vi "Login.vi"() -> ()   [LabVIEW 2020, in "User Lib.lvlib"]
uses:
  User Lib.lvlib
  Database Lib.lvlib
panel:
  out "Error out 2":errorcluster
  out "Error out":errorcluster
  in  "Remember Me":bool
  in  "Cancel":bool
  in  "OK":bool
  in  "Password":string
  in  "Username":string
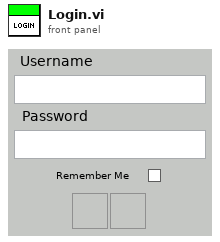
[diagram p1: front panel]
types:
  T1 = cluster{"date/time string":string, "date/time string":string, "code":i32, "date/time string":string, "source":string}
  T2 = cluster{i16, "date/time string":string, "date/time string":string, "Value":string, "Value":string}
  T3 = cluster{i32, "date/time string":string, "date/time string":string, string}
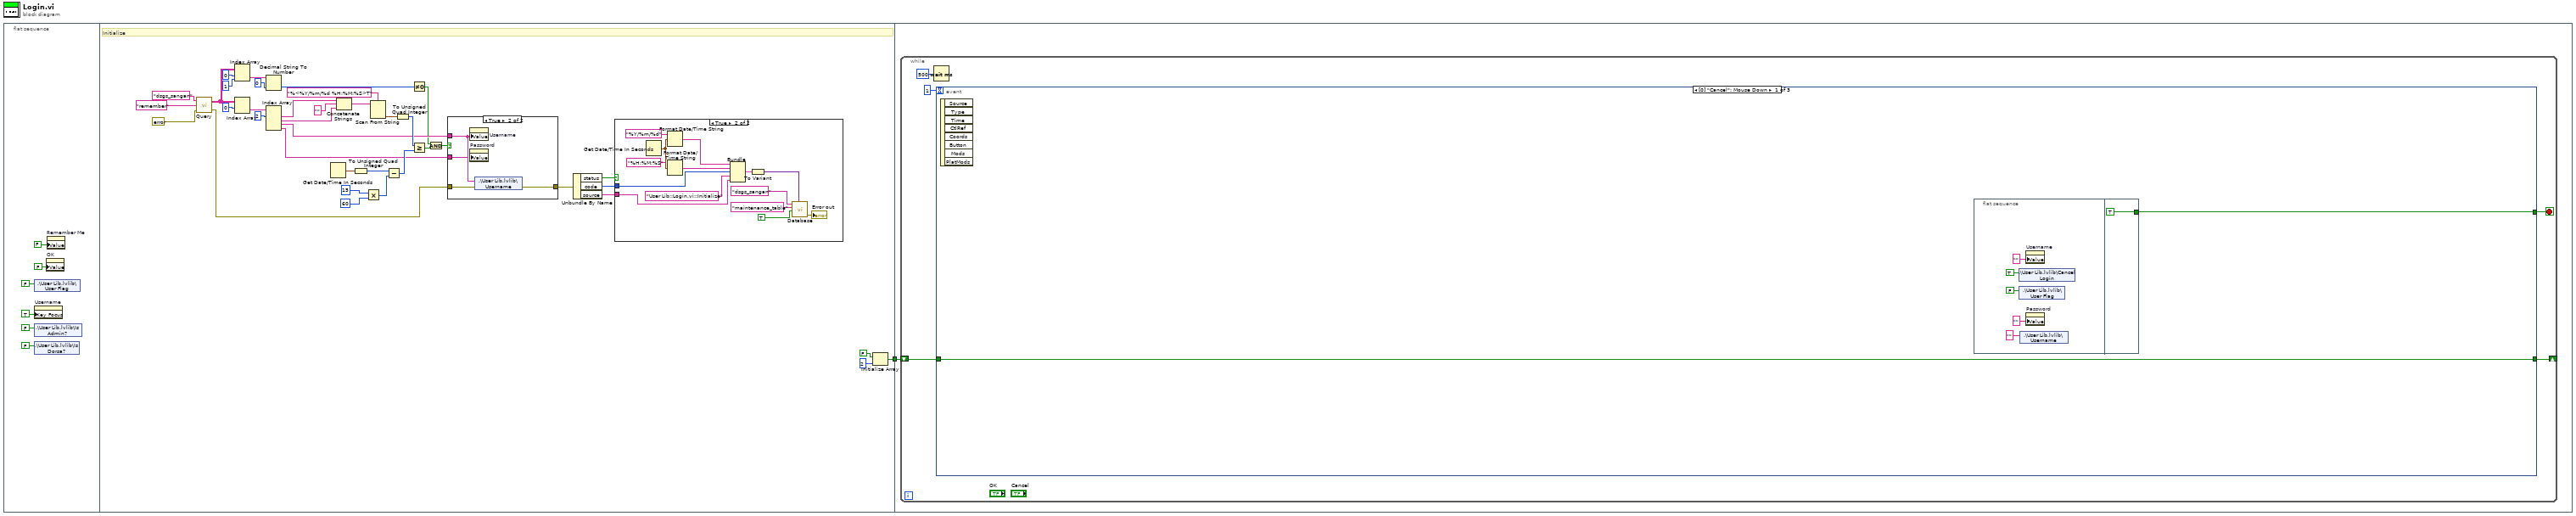
[diagram p0: block diagram]
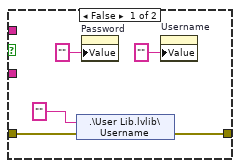
[diagram p3: hidden frame]
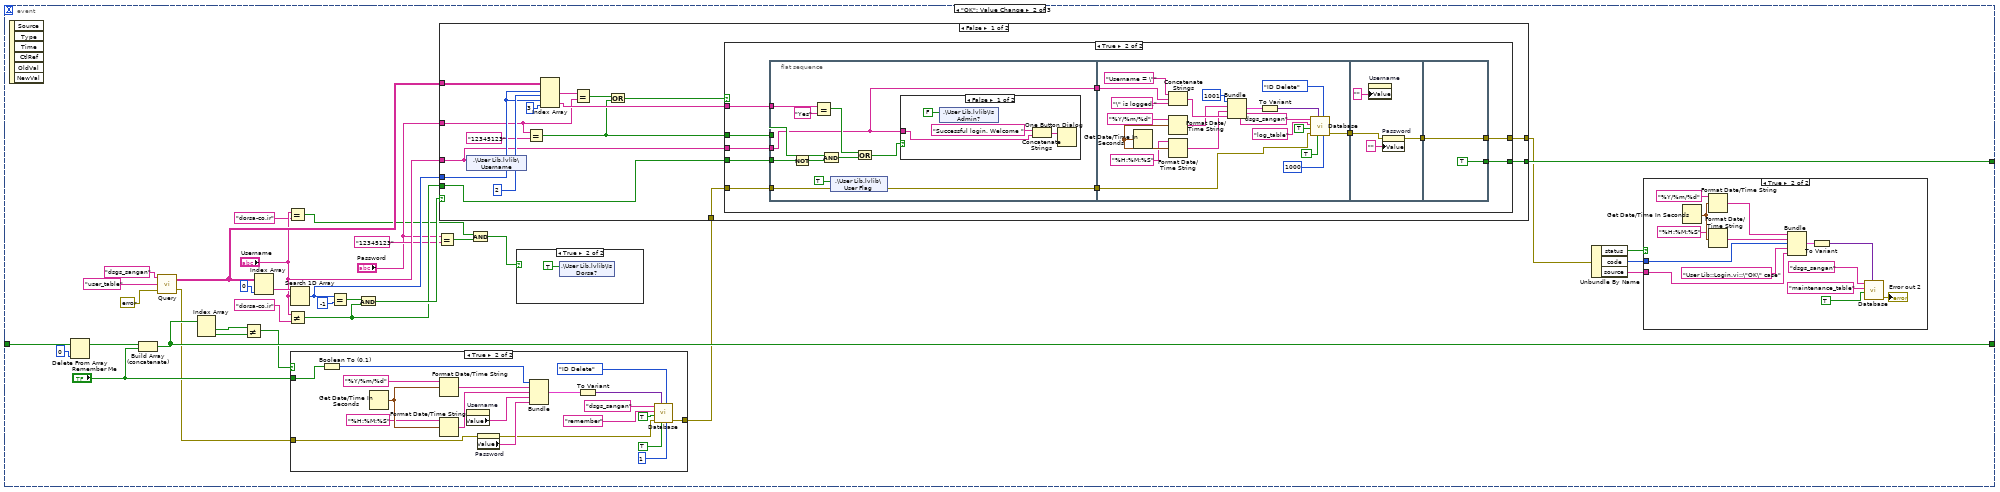
[diagram p4: hidden frame]
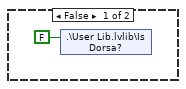
[diagram p7: hidden frame]
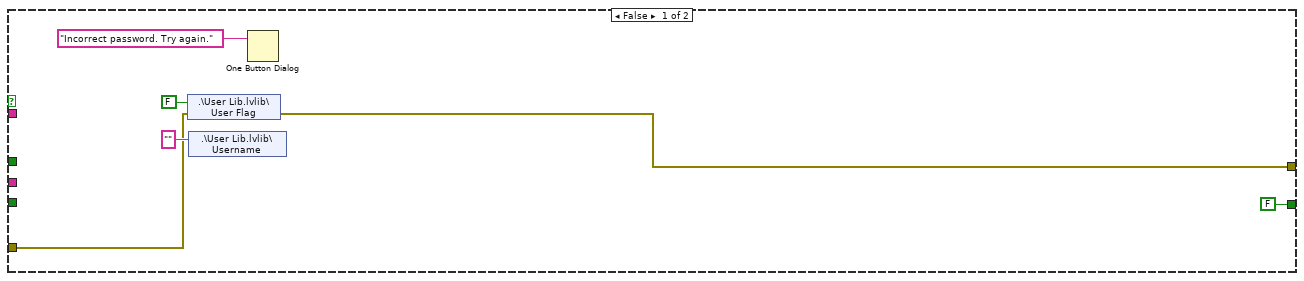
[diagram p8: hidden frame]
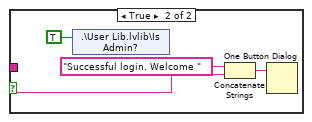
[diagram p9: hidden frame]
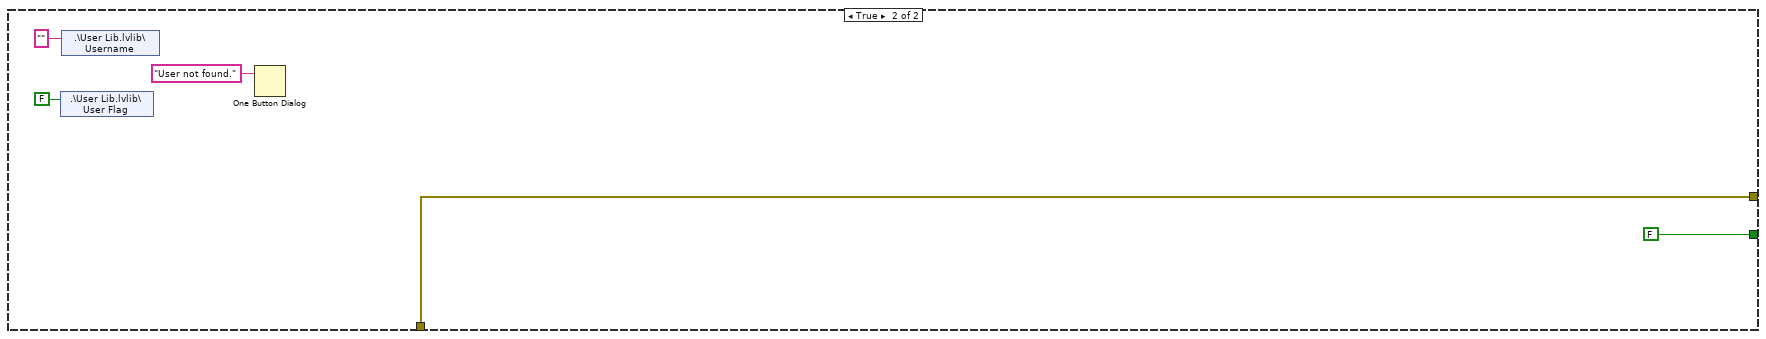
[diagram p10: hidden frame]
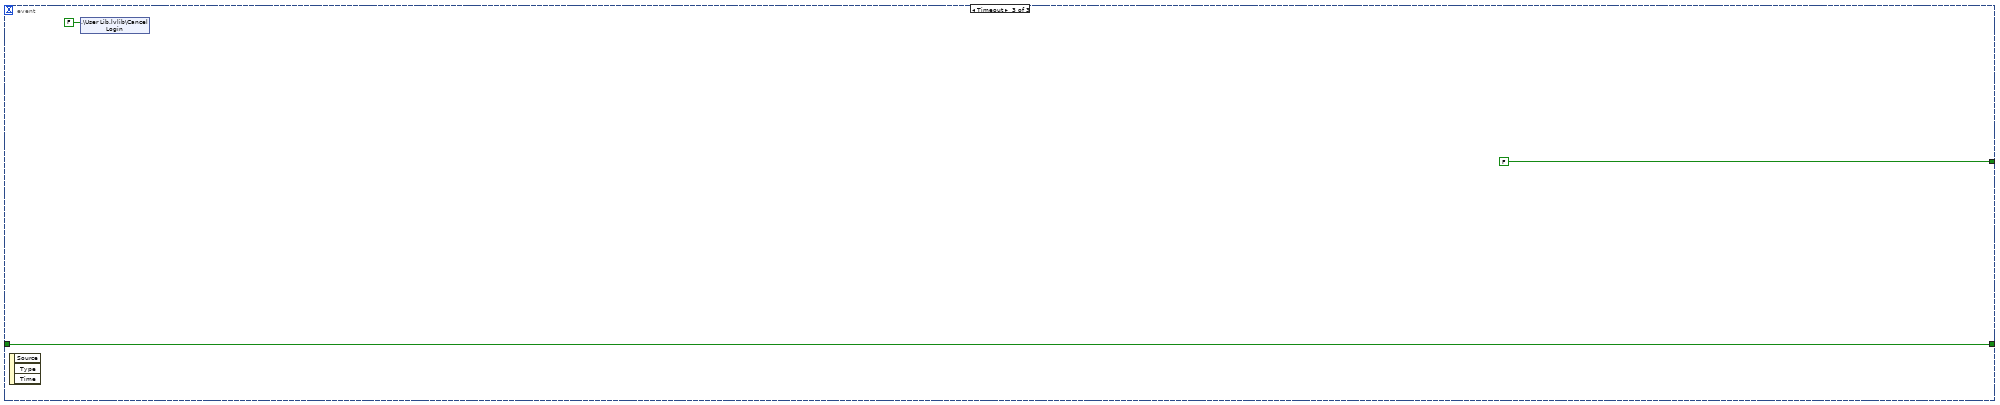
[diagram p11: hidden frame]
diagram:
  n1 = flat-sequence {
    tunnel: [w45] -> w1
    tunnel: w1 -> [w69]
    frame #0 {
      n2 = shared-variable ".\\User Lib.lvlib\\User Flag"(FALSE ("User Flag")) -> ()  [unwired: 1 in, 1 out]
      n3 = property on="Username" class="Str"("Key Focus"=TRUE) -> ()  [unwired: 2 in, 2 out]
      n4 = shared-variable ".\\User Lib.lvlib\\Is Admin?"(FALSE ("Is Admin?")) -> ()  [unwired: 1 in, 1 out]
      n5 = shared-variable ".\\User Lib.lvlib\\Is Dorsa?"(FALSE ("Is Dorsa?")) -> ()  [unwired: 1 in, 1 out]
      n6 = property on="OK" class="Bool"("Value"=FALSE ("OK")) -> ()  [unwired: 2 in, 2 out]
      n7 = property on="Remember Me" class="Bool (strict)"("Value"=FALSE ("Remember Me")) -> ()  [unwired: 2 in, 2 out]
    }
    frame #1 {
      # "Initialize"
      n8 = call "Query.vi"("Error in"=errorcluster {"status"=FALSE, "code"=0, "source"=""}, "Table Name"="remember", "Connection Name"="dsgs_sangan") -> ("Error out"=w11:errorcluster, "data"=w35:string[][])  [unwired: 1 in]
      n9 = Index Array(array=w35, index (row)=0, index (col)=1 ("disabled index (col)")) -> (element=w39:string)
      n10 = Index Array(array=w35, index (row)=0) -> (element=w34:string[])  [unwired: 1 in]
      n11 = Decimal String To Number(string=w39, default (0L)=u8 0 ("default (0 I32)")) -> (number=w37:u8)  [unwired: 1 in, 1 out]
      n12 = Index Array(array=w34, index #1=2 ("index")) -> (element #1=w31:string, element #2=w29:string, element #3=w22:string, element #4=w21:string)  [unwired: 3 in]
      n13 = Get Date/Time In Seconds() -> (seconds since 1Jan1904=w27:timestamp)
      n14 = Concatenate Strings(w31, "" ("string"), w29) -> (w28:string)
      n15 = To Unsigned Quad Integer(1:w27) -> (0:w26:u64)
      n16 = Multiply(x=u64 15 ("y"), y=u64 60) -> (x*y=w8:u64)
      n17 = Scan From String(format string="%<%Y/%m/%d %H:%M:%S>T", input string=w28) -> (output 1=w25:timestamp)  [unwired: 3 in, 3 out]
      n18 = Subtract(x=w26, y=w8) -> (x-y=w23:u64)
      n19 = To Unsigned Quad Integer(1:w25) -> (0:w24:u64)
      n20 = Not Equal To 0?(x=w37) -> (x != 0?=w18:bool)
      n21 = Greater Or Equal?(x=w24, y=w23) -> (x >= y?=w19:bool)
      n22 = And(x=w18, y=w19) -> (x .and. y?=w20:bool)
      n23 = case shown="True" w20 {
        tunnel: w22 -> [_ w68]
        tunnel: w21 -> [_ w67]
        tunnel: w11 -> [w61 w66]
        tunnel: [w60 w65] -> w13
        frame False {
          n24 = shared-variable ".\\User Lib.lvlib\\Username"("" ("Username"), error in=w61) -> (error out=w60:errorcluster)
          n25 = property on="Password" class="Str"("Value"="" ("Password")) -> ()  [unwired: 2 in, 2 out]
          n26 = property on="Username" class="Str"("Value"="" ("Username")) -> ()  [unwired: 2 in, 2 out]
        }
        frame True {
          n27 = property on="Username" class="Str"("Value"=w68) -> ()  [unwired: 2 in, 2 out]
          n28 = property on="Password" class="Str"("Value"=w67) -> ()  [unwired: 2 in, 2 out]
          n29 = shared-variable ".\\User Lib.lvlib\\Username"(w68, error in=w66) -> (error out=w65:errorcluster)
        }
      }
      n30 = Unbundle By Name(w13) -> ("status"=w15:bool, "code"=w16:i32, "source"=w14:string)
      n31 = case shown="True" w15 {
        tunnel: w16 -> [_ w54]
        tunnel: w14 -> [_ w52]
        frame False {
        }
        frame True {
          n32 = Get Date/Time In Seconds() -> (seconds since 1Jan1904=w59:timestamp)
          n33 = Format Date/Time String(time format string (%c)="%Y/%m/%d", seconds (now)=w59) -> (date/time string=w56:string)  [unwired: 1 in]
          n34 = Format Date/Time String(time format string (%c)="%H:%M:%S", seconds (now)=w59) -> (date/time string=w55:string)  [unwired: 1 in]
          n35 = Bundle("date/time string"=w56, "date/time string"=w55, "code"=w54, "date/time string"="User Lib::Login.vi::Initialize", "source"=w52) -> (w51:T1)  [unwired: 1 in]
          n36 = To Variant(anything=w51) -> (Variant=w50:variant)
          n37 = call "Database.vi"("Data"=w50, "Auto Increment ID?"=TRUE, "Table"="maintenance_table", "Connection"="dsgs_sangan") -> ("Error out"=→"Error out":errorcluster)  [unwired: 7 in]
        }
      }
      n38 = Initialize Array(FALSE ("element"), 2 ("dimension size")) -> (w45:bool[])
    }
    frame #2 {
      n39 = while {
        shift-right: [w70] -> _
        shift-left: w69 -> [w71]
        stop <- w72 stop-if-true
        n40 = Wait (ms)(milliseconds to wait=u32 500) -> ()  [unwired: 1 out]
        n41 = event shown="[0] \"Cancel\": Mouse Down" {
          selector: _ -> [_ _ _]
          dyn-events: _ -> [_ _ _]
          timeout: 1 -> [_ _ _]
          tunnel: [w76 w98 FALSE] -> w72
          tunnel: w71 -> [w75 w97 w238]
          tunnel: [w75 w93 w238] -> w70
          event "Cancel": Mouse Down {
            n42 = event-data() -> ()  [unwired: 1 in, 8 out]
            n43 = flat-sequence {
              tunnel: [TRUE] -> w76
              frame #0 {
                n44 = shared-variable ".\\User Lib.lvlib\\Cancel Login"(TRUE ("Login Boolean")) -> ()  [unwired: 1 in, 1 out]
                n45 = shared-variable ".\\User Lib.lvlib\\User Flag"(FALSE ("User Flag")) -> ()  [unwired: 1 in, 1 out]
                n46 = shared-variable ".\\User Lib.lvlib\\Username"("" ("Username")) -> ()  [unwired: 1 in, 1 out]
                n47 = property on="Username" class="Str"("Value"="" ("Username")) -> ()  [unwired: 2 in, 2 out]
                n48 = property on="Password" class="Str"("Value"="" ("Password")) -> ()  [unwired: 2 in, 2 out]
              }
              frame #1 {
              }
            }
          }
          event "OK": Value Change {
            n49 = event-data() -> ()  [unwired: 1 in, 6 out]
            n50 = Delete From Array(array=w97, index=0) -> (array with subset deleted=w95:bool[])  [unwired: 1 in, 1 out]
            n51 = Build Array (concatenate)(w95, "Remember Me") -> (w93:bool[])
            n52 = call "Query.vi"("Error in"=errorcluster {"status"=FALSE, "code"=0, "source"=""}, "Table Name"="user_table", "Connection Name"="dsgs_sangan") -> ("Error out"=w89:errorcluster, "data"=w110:string[][])  [unwired: 1 in]
            n53 = Index Array(array=w93) -> (element #1=w91:bool, element #2=w92:bool)  [unwired: 2 in]
            n54 = Not Equal?(x=w91, y=w92) -> (x != y?=w90:bool)
            n55 = Index Array(array=w110, index (col)=0 ("disabled index (col)")) -> (element=w115:string[])  [unwired: 1 in]
            n56 = Equal?(x="Username", y="dorsa-co.ir") -> (x = y?=w101:bool)
            n57 = Not Equal?(x="Username", y="dorsa-co.ir") -> (x != y?=w106:bool)
            n58 = Search 1D Array(1D array=w115, element="Username") -> (index of element=w113:i32)  [unwired: 1 in]
            n59 = case shown="True" w90 {
              tunnel: "Remember Me" -> [_ w136]
              tunnel: w89 -> [w131 w133]
              tunnel: [w131 w132] -> w87
              frame False {
              }
              frame True {
                n60 = Boolean To (0,1)(Boolean=w136) -> (0, 1=w135:i16)
                n61 = Get Date/Time In Seconds() -> (seconds since 1Jan1904=w144:timestamp)
                n62 = Format Date/Time String(time format string (%c)="%Y/%m/%d", seconds (now)=w144) -> (date/time string=w141:string)  [unwired: 1 in]
                n63 = Format Date/Time String(time format string (%c)="%H:%M:%S", seconds (now)=w144) -> (date/time string=w140:string)  [unwired: 1 in]
                n64 = property on="Username" class="Str"() -> ("Value"=w138:string)  [unwired: 2 in, 2 out]
                n65 = property on="Password" class="Str"(error in=w133) -> (error out=w134:errorcluster, "Value"=w137:string)  [unwired: 1 in, 1 out]
                n66 = Bundle(w135, "date/time string"=w141, "date/time string"=w140, "Value"=w138, "Value"=w137) -> (w139:T2)  [unwired: 1 in]
                n67 = To Variant(anything=w139) -> (Variant=w151:variant)
                n68 = call "Database.vi"("Maximum Row"=1, "Enum"=enum16{"ID Delete", "Time Delete"}."ID Delete", "Delete row?"=TRUE, "Data"=w151, "Error in"=w134, "Auto Increment ID?"=TRUE, "Table"="remember", "Connection"="dsgs_sangan") -> ("Error out"=w132:errorcluster)  [unwired: 3 in]
              }
            }
            n69 = Equal?(x=w113, y=-1) -> (x = y?=w108:bool)
            n70 = And(x=w108, y=w106) -> (x .and. y?=w107:bool)
            n71 = Equal?(x="Password", y="12345123") -> (x = y?=w100:bool)
            n72 = case shown="False" w107 {
              tunnel: w110 -> [w169 _]
              tunnel: w113 -> [w165 _]
              tunnel: "Password" -> [w160 _]
              tunnel: "Username" -> [w157 _]
              tunnel: w106 -> [w159 _]
              tunnel: [w156 FALSE] -> w98
              tunnel: w87 -> [w155 w233]
              tunnel: [w154 w233] -> w83
              frame False {
                n73 = shared-variable ".\\User Lib.lvlib\\Username"(w157) -> ()  [unwired: 1 in, 1 out]
                n74 = Equal?(x=w160, y="12345123" ("x")) -> (x = y?=w158:bool)
                n75 = Index Array(array=w169, index (row) #1=w165, index (col) #1=2 ("disabled index (col)"), index (row) #2=w165, index (col) #2=3 ("index (col)")) -> (element #1=w167:string, element #2=w164:string)
                n76 = Equal?(x=w167, y=w160) -> (x = y?=w163:bool)
                n77 = Or(x=w163, y=w158) -> (x .or. y?=w162:bool)
                n78 = case shown="True" w162 {
                  tunnel: w164 -> [_ w186]
                  tunnel: w159 -> [_ w185]
                  tunnel: w158 -> [_ w184]
                  tunnel: w157 -> [_ w183]
                  tunnel: [FALSE w181] -> w156
                  tunnel: w155 -> [w171 w180]
                  tunnel: [w170 w177] -> w154
                  frame False {
                    n79 = shared-variable ".\\User Lib.lvlib\\User Flag"(FALSE ("User Flag"), error in=w171) -> (error out=w170:errorcluster)
                    n80 = shared-variable ".\\User Lib.lvlib\\Username"("" ("Username")) -> ()  [unwired: 1 in, 1 out]
                    n81 = One Button Dialog(message="Incorrect password. Try again.") -> ()  [unwired: 1 in, 1 out]
                  }
                  frame True {
                    n82 = flat-sequence {
                      tunnel: w186 -> [w196]
                      tunnel: w185 -> [w191]
                      tunnel: w184 -> [w195]
                      tunnel: w183 -> [w189]
                      tunnel: [w189] -> w182
                      tunnel: w180 -> [w188]
                      tunnel: [w187] -> w179
                      tunnel: w182 -> [w211]
                      tunnel: w179 -> [w208]
                      tunnel: [w209] -> w178
                      tunnel: w178 -> [w228]
                      tunnel: [w227] -> w176
                      tunnel: [TRUE] -> w181
                      tunnel: [w231] -> w177
                      tunnel: w176 -> [w231]
                      frame #0 {
                        n83 = Not(x=w191) -> (.not. x?=w190:bool)
                        n84 = Equal?(x=w196, y="Yes") -> (x = y?=w194:bool)
                        n85 = And(x=w195, y=w190) -> (x .and. y?=w193:bool)
                        n86 = shared-variable ".\\User Lib.lvlib\\User Flag"(TRUE, error in=w188) -> (error out=w187:errorcluster)
                        n87 = Or(x=w194, y=w193) -> (x .or. y?=w192:bool)
                        n88 = case shown="False" w192 {
                          tunnel: w189 -> [w200 w204]
                          frame False {
                            n89 = shared-variable ".\\User Lib.lvlib\\Is Admin?"(FALSE ("Is Admin?")) -> ()  [unwired: 1 in, 1 out]
                            n90 = Concatenate Strings("Successful login. Welcome " ("message"), w200) -> (w199:string)
                            n91 = One Button Dialog(message=w199) -> ()  [unwired: 1 in, 1 out]
                          }
                          frame True {
                            n92 = shared-variable ".\\User Lib.lvlib\\Is Admin?"(TRUE ("Is Admin?")) -> ()  [unwired: 1 in, 1 out]
                            n93 = Concatenate Strings("Successful login. Welcome " ("message"), w204) -> (w203:string)
                            n94 = One Button Dialog(message=w203) -> ()  [unwired: 1 in, 1 out]
                          }
                        }
                      }
                      frame #1 {
                        n95 = Get Date/Time In Seconds() -> (seconds since 1Jan1904=w225:timestamp)
                        n96 = Concatenate Strings("Username = \"" ("string"), w211, "\" is logged." ("string")) -> (w226:string)
                        n97 = Format Date/Time String(time format string (%c)="%Y/%m/%d", seconds (now)=w225) -> (date/time string=w224:string)  [unwired: 1 in]
                        n98 = Format Date/Time String(time format string (%c)="%H:%M:%S", seconds (now)=w225) -> (date/time string=w223:string)  [unwired: 1 in]
                        n99 = Bundle(1001, "date/time string"=w224, "date/time string"=w223, w226) -> (w222:T3)  [unwired: 1 in]
                        n100 = To Variant(anything=w222) -> (Variant=w221:variant)
                        n101 = call "Database.vi"("Maximum Row"=1000, "Enum"=enum16{"ID Delete", "Time Delete"}."ID Delete", "Delete row?"=TRUE, "Data"=w221, "Error in"=w208, "Auto Increment ID?"=TRUE, "Table"="log_table" ("table"), "Connection"="dsgs_sangan" ("table")) -> ("Error out"=w209:errorcluster)  [unwired: 3 in]
                      }
                      frame #2 {
                        n102 = property on="Username" class="Str"("Value"="" ("Username")) -> ()  [unwired: 2 in, 2 out]
                        n103 = property on="Password" class="Str"(error in=w228, "Value"="" ("Password")) -> (error out=w227:errorcluster)  [unwired: 1 in, 1 out]
                      }
                      frame #3 {
                      }
                    }
                  }
                }
              }
              frame True {
                n104 = shared-variable ".\\User Lib.lvlib\\User Flag"(FALSE ("User Flag")) -> ()  [unwired: 1 in, 1 out]
                n105 = shared-variable ".\\User Lib.lvlib\\Username"("" ("Username")) -> ()  [unwired: 1 in, 1 out]
                n106 = One Button Dialog(message="User not found.") -> ()  [unwired: 1 in, 1 out]
              }
            }
            n107 = And(x=w101, y=w100) -> (x .and. y?=w99:bool)
            n108 = case shown="True" w99 {
              frame False {
                n109 = shared-variable ".\\User Lib.lvlib\\Is Dorsa?"(FALSE ("Is Dorsa?")) -> ()  [unwired: 1 in, 1 out]
              }
              frame True {
                n110 = shared-variable ".\\User Lib.lvlib\\Is Dorsa?"(TRUE ("Is Dorsa?")) -> ()  [unwired: 1 in, 1 out]
              }
            }
            n111 = Unbundle By Name(w83) -> ("status"=w85:bool, "code"=w86:i32, "source"=w84:string)
            n112 = case shown="True" w85 {
              tunnel: w86 -> [_ w125]
              tunnel: w84 -> [_ w123]
              frame False {
              }
              frame True {
                n113 = Get Date/Time In Seconds() -> (seconds since 1Jan1904=w130:timestamp)
                n114 = Format Date/Time String(time format string (%c)="%Y/%m/%d", seconds (now)=w130) -> (date/time string=w127:string)  [unwired: 1 in]
                n115 = Format Date/Time String(time format string (%c)="%H:%M:%S", seconds (now)=w130) -> (date/time string=w126:string)  [unwired: 1 in]
                n116 = Bundle("date/time string"=w127, "date/time string"=w126, "code"=w125, "date/time string"="User Lib::Login.vi::\"OK\" case", "source"=w123) -> (w122:T1)  [unwired: 1 in]
                n117 = To Variant(anything=w122) -> (Variant=w121:variant)
                n118 = call "Database.vi"("Data"=w121, "Auto Increment ID?"=TRUE, "Table"="maintenance_table", "Connection"="dsgs_sangan") -> ("Error out"=→"Error out 2":errorcluster)  [unwired: 7 in]
              }
            }
          }
          event Timeout {
            n119 = event-data() -> ()  [unwired: 1 in, 3 out]
            n120 = shared-variable ".\\User Lib.lvlib\\Cancel Login"(FALSE ("Login Boolean")) -> ()  [unwired: 1 in, 1 out]
          }
        }
      }
    }
  }
